vi "Remove_call_chain.vi"(0 "Error Description":string) -> (4 "Description Without Call Chain":string)   [LabVIEW 2020]
doc: "This Subvi is used to remove the call chain from the error description."
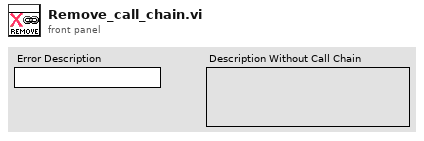
[diagram p1: front panel]
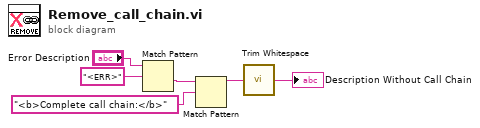
[diagram p0: block diagram]
diagram:
  n1 = Match Pattern(string="Error Description", regular expression="<ERR>") -> (after substring=w2:string)  [unwired: 1 in, 3 out]
  n2 = Match Pattern(string=w2, regular expression="<b>Complete call chain:</b>") -> (before substring=w1:string)  [unwired: 1 in, 3 out]
  n3 = call <vilib>:"Trim Whitespace.vi"("string"=w1) -> ("trimmed string"=→"Description Without Call Chain":string)  [unwired: 1 in]
